vi "Bairstow_Quadratic Roots.vi"(11 "quadratic":dbl[](array[numeric]) format="%#.6g") -> (2 "Complex Pair Roots":cdb[](array[numeric]) format="%#.6g", 3 "Real Roots":dbl[](array[numeric]))   [LabVIEW 2018, in "NI_AALPro.lvlib"]
uses:
  NI_AALPro.lvlib
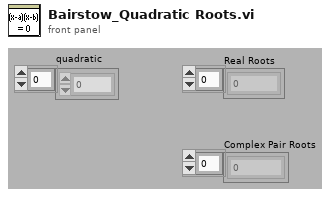
[diagram p1: front panel]
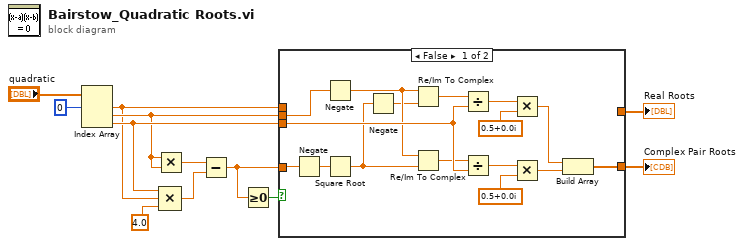
[diagram p0: block diagram]
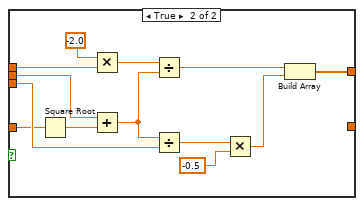
[diagram p2: hidden frame]
diagram:
  n1 = Index Array(array="quadratic", index #1=0 ("index")) -> (element #1=w3:dbl, element #2=w4:dbl, element #3=w6:dbl)  [unwired: 2 in]
  n2 = Multiply(x=w4, y=w4) -> (x*y=w10:dbl)
  n3 = Compound Arithmetic op=MULTIPLY(w6, w3, 4.0) -> (w9:dbl)
  n4 = Subtract(x=w10, y=w9) -> (x-y=w7:dbl)
  n5 = Greater Or Equal To 0?(x=w7) -> (x >= 0?=w8:bool)
  n6 = case shown="False" w8 {
    tunnel: w7 -> [w28 w32]
    tunnel: w4 -> [w26 w41]
    tunnel: w6 -> [w25 w36]
    tunnel: w3 -> [_ w40]
    tunnel: [_ w29] -> w1
    tunnel: [w13 _] -> w2
    frame False {
      n7 = Negate(x=w28) -> (-x=w27:dbl)
      n8 = Negate(x=w26) -> (-x=w20:dbl)
      n9 = Square Root(x=w27) -> (sqrt(x)=w17:dbl)
      n10 = Negate(x=w17) -> (-x=w18:dbl)
      n11 = Re/Im To Complex(1:w18, 2:w20) -> (0:w19:cdb)
      n12 = Re/Im To Complex(1:w17, 2:w20) -> (0:w16:cdb)
      n13 = Divide(x=w19, y=w25) -> (x/y=w24:cdb)
      n14 = Divide(x=w16, y=w25) -> (x/y=w22:cdb)
      n15 = Multiply(x=w24, y=cdb 0.5+0.0i) -> (x*y=w15:cdb)
      n16 = Multiply(x=w22, y=cdb 0.5+0.0i) -> (x*y=w14:cdb)
      n17 = Build Array(w15, w14) -> (w13:cdb[])
    }
    frame True {
      n18 = Square Root(x=w32) -> (sqrt(x)=w33:dbl)
      n19 = Multiply(x=-2.0, y=w40) -> (x*y=w38:dbl)
      n20 = Add(x=w41, y=w33) -> (x+y=w37:dbl)
      n21 = Divide(x=w38, y=w37) -> (x/y=w30:dbl)
      n22 = Divide(x=w37, y=w36) -> (x/y=w35:dbl)
      n23 = Multiply(x=w35, y=-0.5 ("x")) -> (x*y=w31:dbl)
      n24 = Build Array(w30, w31) -> (w29:dbl[])
    }
  }
  "Complex Pair Roots" <- w2
  "Real Roots" <- w1
